vi "Display Settings.vi"(8 "error in (no error)":errorcluster, 11 "Fixture in":refnum<class "Fixture.lvclass">) -> (0 "error out":errorcluster, 2 "Settings":i32[](array[numeric]), 3 "Fixture out":refnum<class "Fixture.lvclass">)   [LabVIEW 2016, in "Fixture.lvclass"]
uses:
  Fixture.lvclass
  Fixture.lvclass/Fixture.ctl
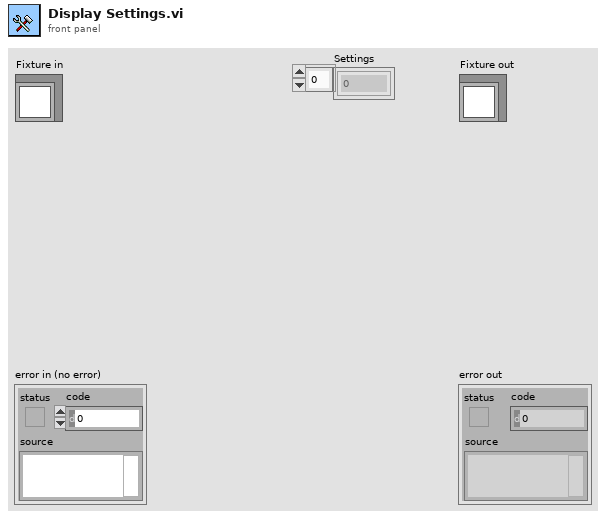
[diagram p1: front panel]
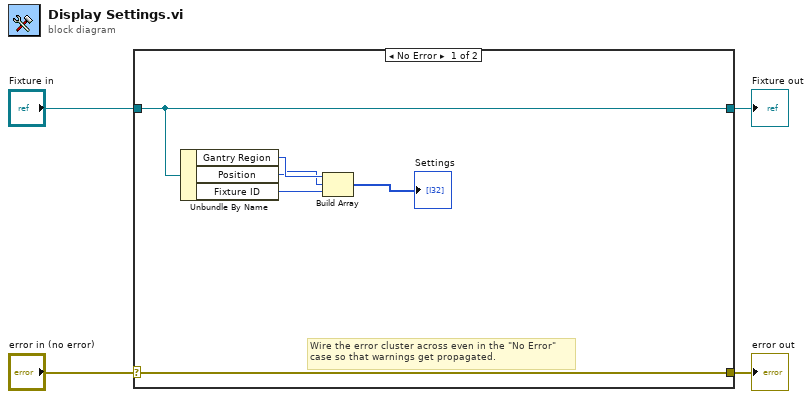
[diagram p0: block diagram]
diagram:
  n1 = case shown="No Error" "error in (no error)" {
    selector: "error in (no error)" -> [w10 w12]
    tunnel: [w10 w12] -> w3
    tunnel: [w9 w11] -> w1
    tunnel: "Fixture in" -> [w9 w11]
    frame No Error {
      # "Wire the error cluster across even in the \"No Error\"\ncase so that warnings get propagated."
      n2 = Unbundle By Name(w9) -> ("Gantry Region"=w8:i32, "Position"=w7:i32, "Fixture ID"=w6:i32)
      n3 = Build Array(w8, w7, w6) -> (→"Settings":i32[])
    }
    frame Error {
    }
  }
  "error out" <- w3
  "Fixture out" <- w1
